vi "baseline_sub1.vi"(7 "x 2":dbl, 8 "x 3":dbl, 9 "Boolean":bool, 10 "data":dbl[](array[numeric])) -> (1 "X":dbl[](array[numeric]), 3 "Y":dbl[](array[numeric]))   [LabVIEW 2015]
uses:
  <vilib>/Analysis/baseanly.llb/Mean (DBL).vi
  <vilib>/Analysis/NI_AALBase.lvlib
  <vilib>/Analysis/NI_AALPro.lvlib
panel:
  out "Waveform Graph":dynamicdata(graph)
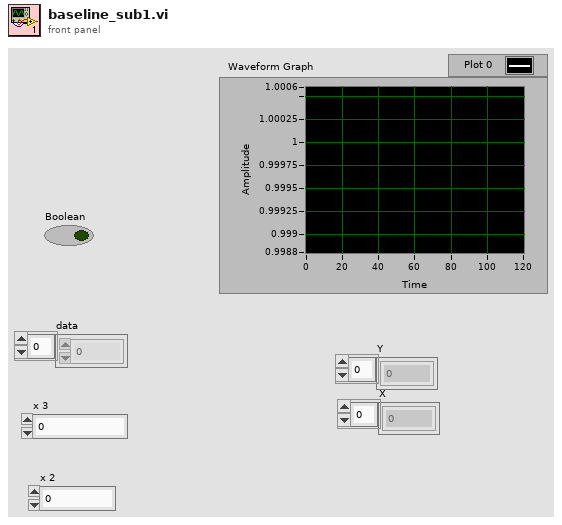
[diagram p1: front panel]
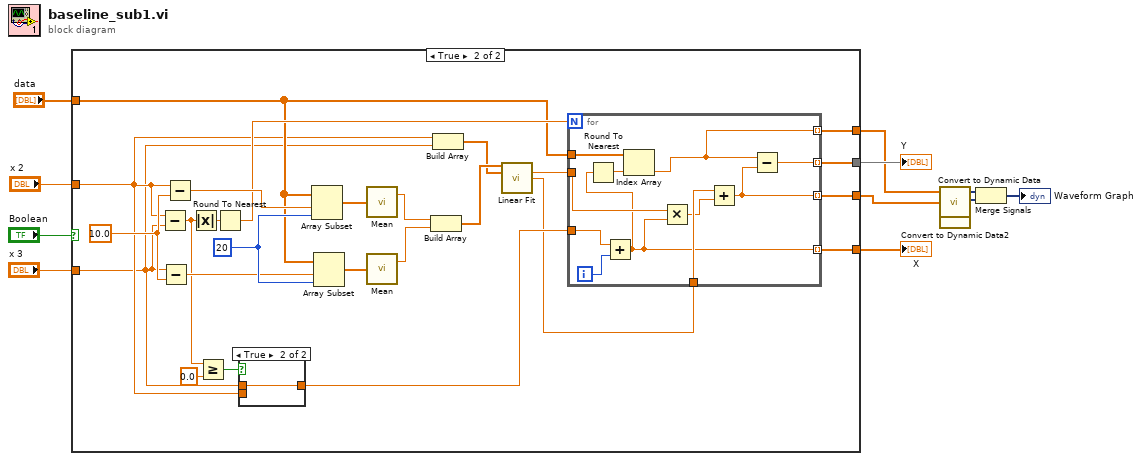
[diagram p0: block diagram]
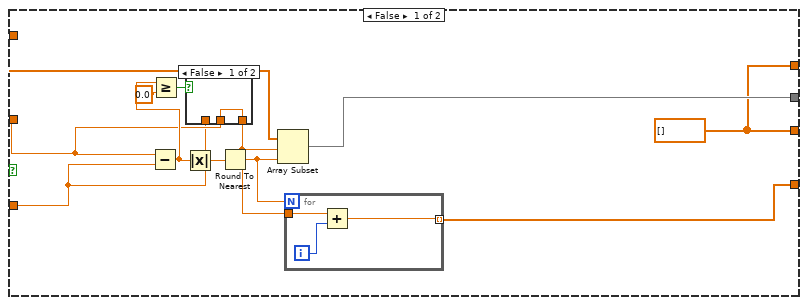
[diagram p2: hidden frame]
diagram:
  n1 = case shown="True" "Boolean" {
    tunnel: [w17 w35] -> w6
    tunnel: [w16 w34] -> w7
    tunnel: "data" -> [w13 w33]
    tunnel: "x 2" -> [w15 w32]
    tunnel: "x 3" -> [w14 w31]
    tunnel: [w12 w30] -> w3
    tunnel: [w12 w29] -> w5
    frame False {
      w12 = dbl[] []
      n2 = Subtract(x=w15, y=w14) -> (x-y=w22:dbl)
      n3 = Greater Or Equal?(x=w22, y=0.0) -> (x >= y?=w23:bool)
      n4 = Absolute Value(x=w22) -> (abs(x)=w19:dbl)
      n5 = case shown="False" w23 {
        tunnel: w14 -> [_ w25]
        tunnel: [w24 w25] -> w20
        tunnel: w15 -> [w24 _]
        frame False {
        }
        frame True {
        }
      }
      n6 = Round To Nearest(number=w19) -> (nearest integer value=w18:dbl)
      n7 = Array Subset(array=w13, index=w20, length=w18) -> (w17:dbl[])
      n8 = for {
        N: w18 -> [_]
        tunnel: [w26] -> w16 mode=indexing
        tunnel: w20 -> [w28]
        i -> [w27]
        n9 = Add(x=w28, y=w27) -> (x+y=w26:dbl)
      }
    }
    frame True {
      w52 = 10.0 ("y")
      w53 = 20 ("length")
      n10 = Subtract(x=w32, y=w31) -> (x-y=w39:dbl)
      n11 = Subtract(x=w31, y=w52) -> (x-y=w45:dbl)
      n12 = Subtract(x=w32, y=w52) -> (x-y=w44:dbl)
      n13 = Absolute Value(x=w39) -> (abs(x)=w43:dbl)
      n14 = Greater Or Equal?(x=w39, y=0.0) -> (x >= y?=w41:bool)
      n15 = Round To Nearest(number=w43) -> (nearest integer value=w42:dbl)
      n16 = case shown="True" w41 {
        tunnel: w31 -> [_ w55]
        tunnel: w32 -> [w54 _]
        tunnel: [w54 w55] -> w38
        frame False {
        }
        frame True {
        }
      }
      n17 = Array Subset(array=w33, index=w44, length=w53) -> (w51:dbl[])
      n18 = Array Subset(array=w33, index=w45, length=w53) -> (w50:dbl[])
      n19 = call-poly <vilib>:"Mean.vi"("X"=w51) -> ("mean"=w49:dbl)  [unwired: 1 out]
      n20 = call-poly <vilib>:"Mean.vi"("X"=w50) -> ("mean"=w48:dbl)  [unwired: 1 out]
      n21 = Build Array(w49, w48) -> (w47:dbl[])
      n22 = Build Array(w32, w31) -> (w46:dbl[])
      n23 = call <vilib>:"Linear Fit.vi"("Y"=w47, "X"=w46) -> ("slope"=w37:dbl, "intercept"=w36:dbl)  [unwired: 9 in, 3 out]
      n24 = for {
        N: w42 -> [_]
        tunnel: w38 -> [w64]
        tunnel: [w56] -> w34 mode=indexing
        tunnel: w33 -> [w65]
        tunnel: w37 -> [w62]
        tunnel: w36 -> [w61]
        tunnel: [w59] -> w35 mode=indexing
        tunnel: [w58] -> w30 mode=indexing
        tunnel: [w57] -> w29 mode=indexing
        i -> [w66]
        n25 = Add(x=w64, y=w66) -> (x+y=w56:dbl)
        n26 = Round To Nearest(number=w56) -> (nearest integer value=w63:dbl)
        n27 = Index Array(array=w65, index=w63) -> (element=w57:dbl)
        n28 = Multiply(x=w62, y=w56) -> (x*y=w60:dbl)
        n29 = Add(x=w61, y=w60) -> (x+y=w58:dbl)
        n30 = Subtract(x=w57, y=w58) -> (x-y=w59:dbl)
      }
    }
  }
  "Y" <- w6
  "X" <- w7
  n31 = call "Convert to Dynamic Data"("Array"=w5) -> ("Dynamic Data Type"=w4:dynamicdata)  [unwired: 3 in]
  n32 = call "Convert to Dynamic Data2"("Array"=w3) -> ("Dynamic Data Type"=w2:dynamicdata)  [unwired: 3 in]
  n33 = Merge Signals(w4, w2) -> (→"Waveform Graph":dynamicdata)
